vi "SelectMeterChannel.vi"(2 "ChannelSelection":dbl, 3 "error out":errorcluster, 4 "reference out":refnum<visa-resource-name>) -> (0 "error out 2":errorcluster, 1 "reference out 2":refnum<visa-resource-name>)   [LabVIEW 2009]
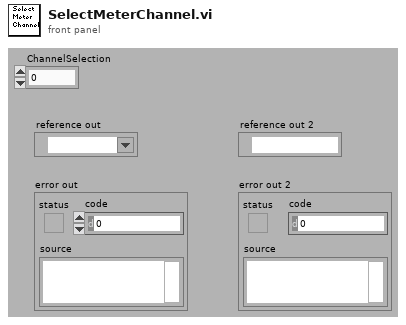
[diagram p1: front panel]
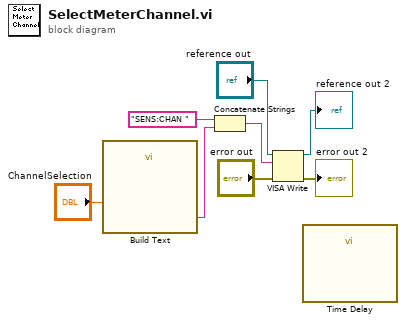
[diagram p0: block diagram]
diagram:
  n1 = call "Build Text"("ChannelSelection"="ChannelSelection") -> ("Result"=w2:string)  [unwired: 13 in, 1 out]
  n2 = Concatenate Strings("SENS:CHAN " ("write buffer"), w2) -> (w1:string)
  n3 = VISA Write(VISA resource name="reference out", write buffer=w1, error in (no error)="error out") -> (VISA resource name out=→"reference out 2":refnum<visa-resource-name>, error out=→"error out 2":errorcluster)  [unwired: 1 out]
  n4 = call "Time Delay"() -> ()  [unwired: 11 in, 1 out]
